vi "Connect.vi"(8 "error in (no error)":errorcluster, 11 "Optris PI in":refnum<class "Optris PI.lvclass">) -> (0 "error out":errorcluster, 3 "Optris PI out":refnum<class "Optris PI.lvclass">)   [LabVIEW 2018, in "Optris PI.lvlib" / "Optris PI.lvclass"]
uses:
  Optris PI.lvclass
  <instrlib>/Optris PI/libirimager_direct_binding.lvlib
  PPLs/Thermal Camera/Parent/Thermal Camera.lvlibp/Thermal Camera.lvclass
  C:/AME Test Engineering/LabVIEW/PPLs/Thermal Camera/Parent/Thermal Camera.lvlibp/Thermal Camera.lvclass
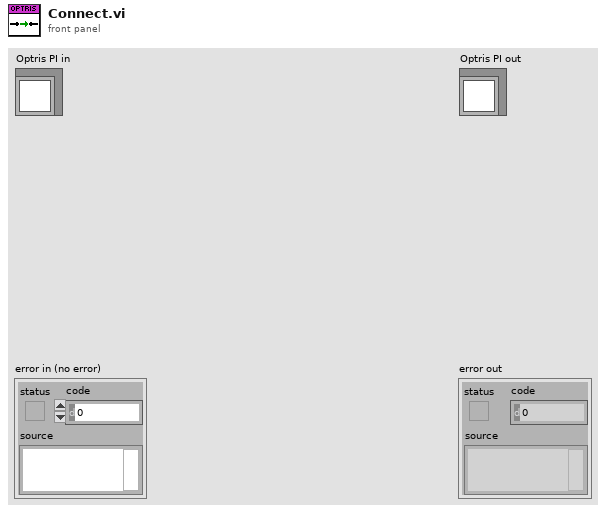
[diagram p1: front panel]
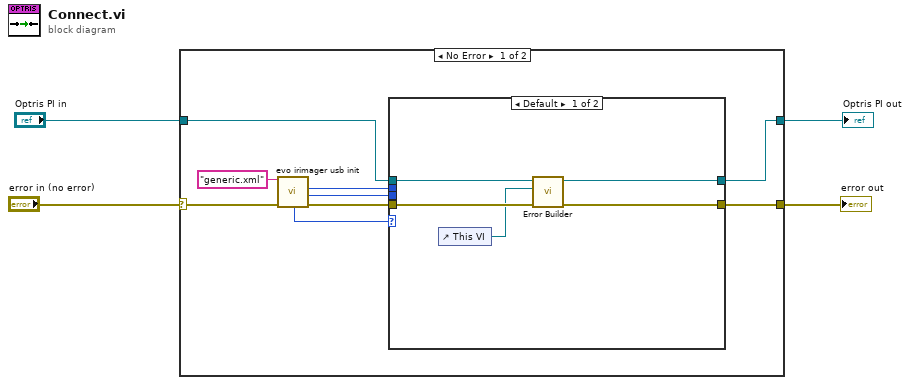
[diagram p0: block diagram]
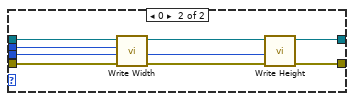
[diagram p2: hidden frame]
diagram:
  n1 = case shown="No Error" "error in (no error)" {
    selector: "error in (no error)" -> [w13 w28]
    tunnel: [w8 w28] -> w3
    tunnel: "Optris PI in" -> [w6 w27]
    tunnel: [w5 w27] -> w1
    frame No Error {
      n2 = call <instrlib>:"evo irimager usb init.vi"("xml_config"="generic.xml", "error in (no error)"=w13) -> ("f(x) return"=w7:i32, "width out"=w11:i32, "height out"=w9:i32, "error out"=w10:errorcluster)  [unwired: 9 in, 1 out]
      n3 = case shown="Default" w7 {
        tunnel: w6 -> [w16 w26]
        tunnel: w11 -> [_ w25]
        tunnel: w10 -> [w18 w24]
        tunnel: w9 -> [_ w22]
        tunnel: [w15 w20] -> w5
        tunnel: [w17 w19] -> w8
        frame Default {
          n4 = control-ref of="This VI"() -> (w14:refnum<vi>)
          n5 = call "Error Builder.vi"("error in (no error)"=w18, "This VI"=w14, "Optris PI in"=w16) -> ("Error out"=w17:errorcluster, "Optris PI out"=w15:refnum<class "Optris PI.lvclass">)  [unwired: 7 in]
        }
        frame 0 {
          n6 = call "Write Width.vi"("error in (no error)"=w24, "Width"=w25, "Thermal Camera in"=w26) -> ("error out"=w21:errorcluster, "Thermal Camera out"=w23:refnum<class "Optris PI.lvclass">)  [unwired: 7 in]
          n7 = call "Write Height.vi"("error in (no error)"=w21, "Height"=w22, "Thermal Camera in"=w23) -> ("error out"=w19:errorcluster, "Thermal Camera out"=w20:refnum<class "Optris PI.lvclass">)  [unwired: 7 in]
        }
      }
    }
    frame Error {
    }
  }
  "error out" <- w3
  "Optris PI out" <- w1
